vi "STM Write Meta.vi"(8 "error in":errorcluster, 10 "Meta data":T1[](array[typedef]), 11 "connection ID":refnum<k5>) -> (0 "error out":errorcluster, 3 "connection ID out":refnum<k5>)   [LabVIEW 2015]
doc: "Use this VI to transmit the Meta data cluster to a remote computer. Sending the meta data to another computers helps maintainability since the data resides only on one side and it is shared to other computers at run time.\n\nThe meta data cluster must contain valid name and type information before being sent.\n\nThis VI converts the meta data cluster into XML format before transfering it to a remote computer. If your application communicates with a non-LabVIEW program, you can still use this VI but make sure the receiving code knows how to parse through the XML string."
uses:
  Data Def/stm_MetaElement.ctl
  Data Def/stm_MetaDataElement.ctl
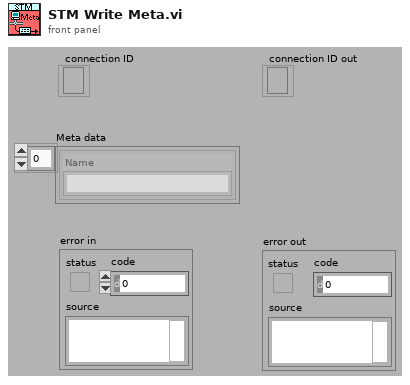
[diagram p1: front panel]
types:
  T1 = typedef "stm_MetaElement.ctl" = cluster{"Name":T2}
  T2 = typedef "stm_MetaDataElement.ctl" = string
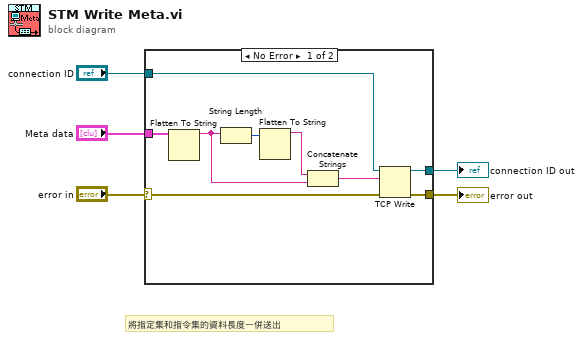
[diagram p0: block diagram]
diagram:
  # "將指定集和指令集的資料長度一併送出"
  n1 = case shown="No Error" "error in" {
    selector: "error in" -> [w10 w16]
    tunnel: [w14 w15] -> w5
    tunnel: "connection ID" -> [w13 w15]
    tunnel: "Meta data" -> [w12 _]
    tunnel: [w11 w16] -> w2
    frame No Error {
      n2 = Flatten To String(anything=w12) -> (data string=w6:string)  [unwired: 1 in, 4 out]
      n3 = String Length(string=w6) -> (length=w9:i32)
      n4 = Flatten To String(anything=w9) -> (data string=w8:string)  [unwired: 1 in, 4 out]
      n5 = Concatenate Strings(w8, w6) -> (w7:string)
      n6 = TCP Write(connection ID=w13, data in=w7, error in (no error)=w10) -> (connection ID out=w14:refnum<k5>, error out=w11:errorcluster)  [unwired: 2 out]
    }
    frame Error {
    }
  }
  "connection ID out" <- w5
  "error out" <- w2
